vi "General Least Squares Fitting.vi"() -> ()   [LabVIEW 2023]
doc: "Determines a generalized linear fit for a set of observed data pairs using the General Linear Fit VI. This example uses a model that is linear function of the coefficients (a0 through an). The model describes the relationship between X and Y as follows.\n\nY fitted = a0* Y0(X)+a1* Y1(X)+...an* Yn(X)\n\nWhere Yi(X) can be a nonlinear function of X observed, and Y fitted is the fitting result."
uses:
  <vilib>/Analysis/1siggen.llb/Ramp Pattern by Samples.vi
  <vilib>/Analysis/NI_AALBase.lvlib
  <vilib>/Analysis/NI_AALPro.lvlib
panel:
  out "Best Fit Model":string
  out "Observed Data and Fitted Curve":T1(graph)
  out "Coefficients":dbl[](array[numeric]) format="%0.4f"
  in  "Noise Amplitude":dbl=2.0
  in  "Number of Points":i32=128 format="%0.0f"
  out "MSE":dbl
  # "Overview: Demonstrates fitting data using a linear combination of basis functions.\nRequirements: LabVIEW Full Development System\nInstructions:\nRun the VI."
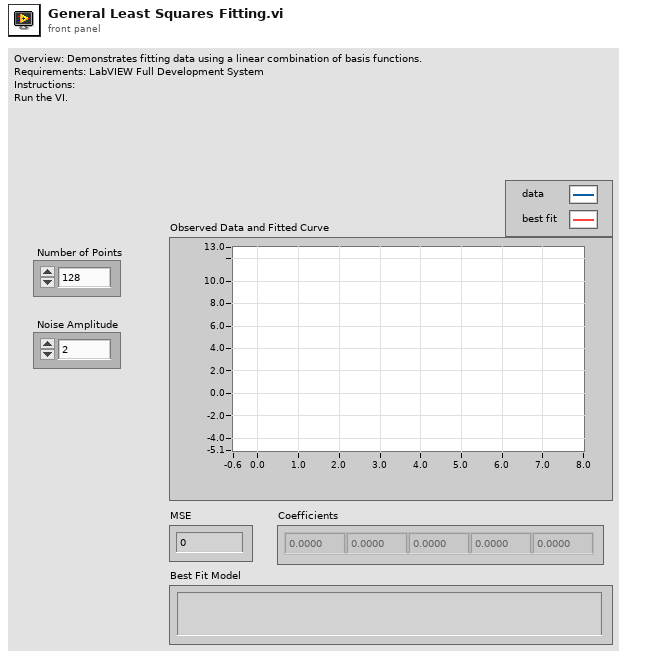
[diagram p1: front panel]
types:
  T1 = cluster{"Ramp Pattern":dbl[], "Best Fit":dbl[]}[]
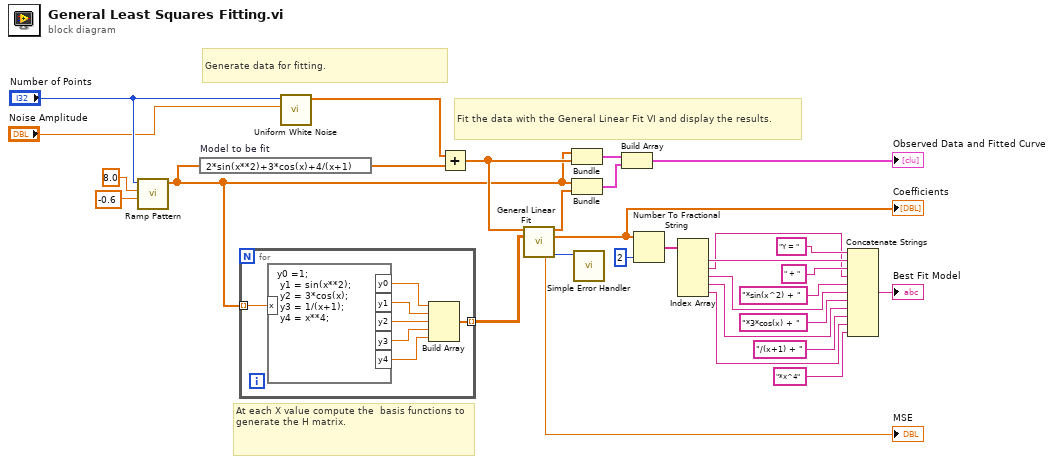
[diagram p0: block diagram]
diagram:
  # "Fit the data with the General Linear Fit VI and display the results."
  # "At each X value compute the  basis functions to generate the H matrix."
  # "Generate data for fitting."
  n1 = call-poly <vilib>:"Ramp Pattern.vi"("start"=-0.6 ("end"), "end"=8.0, "samples"="Number of Points") -> ("Ramp Pattern"=w20:dbl[])  [unwired: 7 in, 1 out]
  n2 = expression code="2*sin(x**2)+3*cos(x)+4/(x+1)" "Model to be fit"(w20) -> (w26:dbl[])
  n3 = for {
    tunnel: w20 -> [w31] mode=indexing
    tunnel: [w33] -> w29 mode=indexing
    n4 = formula code="y0 =1;\n y1 = sin(x**2);\n y2 = 3*cos(x);\n y3 = 1/(x+1);\n y4 = x**4;"("x"=w31) -> ("y4"=w37:dbl, "y3"=w34:dbl, "y2"=w36:dbl, "y1"=w35:dbl, "y0"=w32:dbl)
    n5 = Build Array(w32, w35, w36, w34, w37) -> (w33:dbl[])
  }
  n6 = call <vilib>:"Uniform White Noise.vi"("amplitude"="Noise Amplitude", "samples"="Number of Points") -> ("uniform white noise"=w23:dbl[])  [unwired: 8 in, 1 out]
  n7 = Add(x=w23, y=w26) -> (x+y=w21:dbl[])
  n8 = call <vilib>:"General Linear Fit.vi"("Y"=w21, "H"=w29) -> ("Best Fit"=w19:dbl[], "Coefficients"=w8:dbl[], "residue"=→"MSE":dbl, "error"=w16:i32)  [unwired: 8 in, 2 out]
  "Coefficients" <- w8
  n9 = Bundle("Ramp Pattern"=w20, w21) -> (w22:cluster{"Ramp Pattern":dbl[], dbl[]})  [unwired: 1 in]
  n10 = Bundle("Ramp Pattern"=w20, "Best Fit"=w19) -> (w18:cluster{"Ramp Pattern":dbl[], "Best Fit":dbl[]})  [unwired: 1 in]
  n11 = call <vilib>:"Simple Error Handler.vi"("error code (no error:0)"=w16) -> ()  [unwired: 4 in, 5 out]
  n12 = Build Array(w22, w18) -> (→"Observed Data and Fitted Curve":T1)
  n13 = Number To Fractional String(number=w8, precision (6)=2) -> (F-format string=w11:string[])  [unwired: 2 in]
  n14 = Index Array(array=w11) -> (element #1=w10:string, element #2=w2:string, element #3=w9:string, element #4=w7:string, element #5=w3:string)  [unwired: 5 in]
  n15 = Concatenate Strings("Y = ", w10, " + ", w2, "*sin(x^2) + ", w9, "*3*cos(x) + ", w7, "/(x+1) + ", w3, "*x^4") -> (→"Best Fit Model":string)
